vi "test_fpga_sicm_main.vi"() -> ()   [LabVIEW 2016]
uses:
  <vilib>/Platform/TimedLoop/XDataNode/timing_clust.ctl
  <vilib>/Platform/TimedLoop/XDataNode/nitl_modes.ctl
  <vilib>/Platform/TimedLoop/XDataNode/wakeup.ctl
  <vilib>/rvi/Emulation/niFpgaSctlEmulationGetInTimedLoop.vi
  <vilib>/rvi/Emulation/niFpgaEmulationReportErrorSimple.vi
  <vilib>/rvi/Emulation/niFpgaGetClockAttributes.vi
  <vilib>/rvi/Emulation/niFpgaCriticalErrorInLSC.vi
  <vilib>/Platform/TimedLoop/XDataNode/XDataNode.xnode
  <vilib>/Platform/TimedLoop/XDataNode/XDNodeRunTimeDep.lvlib
panel:
  out "sicm.Baseline":T1
  out "debug":T2
  in  "sicm.p.modes":T3
  in  "sicm.display":cluster{"sicm.ptsAfterTrig":u16}
  out "heightOut":T4
  in  "sicm.p.params":T5={"sicm.p.setPoint"=0.9999847412109375, "sicm.p.setPointFrac"=1.0, "stepDown"=0.0, "retractHeight"=0.0, "adaptiveMin"=0.0} {"sicm.p.setPoint" format="%#_3g"}
  out "sicm.triggerHeight":T6
  in  "sicm.i.current":T7
  in  "sicm.p.clocks":T8
  in  "sicm.blc.p.params":T9={"se.blc.p.postRetractDelay"=0, "se.blc.p.windowSize"=0, "se.blc.p.updateFactor"=-8, "blc.resetBackground"=FALSE}
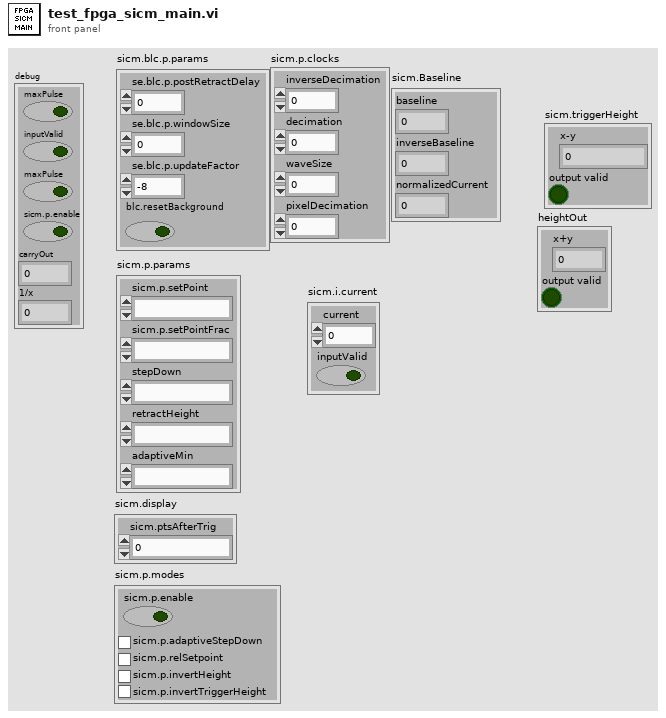
[diagram p1: front panel]
types:
  T1 = cluster{"carryOut":fxp<+/-,22,2>, "1/x":fxp<+/-,32,24>, "normalizedCurrent":fxp<+,20,1>}
  T2 = cluster{"maxPulse":bool, "inputValid":bool, "maxPulse":bool, "sicm.p.enable":bool, "carryOut":fxp<+/-,22,2>, "1/x":fxp<+/-,27,24>}
  T3 = cluster{"sicm.p.enable":bool, "sicm.p.adaptiveStepDown":bool, "sicm.p.relSetpoint":bool, "sicm.p.invertHeight":bool, "sicm.p.invertTriggerHeight":bool}
  T4 = cluster{"x+y":fxp<+/-,28,2>, "output valid":bool}
  T5 = cluster{"sicm.p.setPoint":fxp<+,20,0>, "sicm.p.setPointFrac":fxp<+/-,20,14>, "stepDown":fxp<+/-,28,4>, "retractHeight":fxp<+/-,28,4>, "adaptiveMin":fxp<+,10,0>}
  T6 = cluster{"x-y":fxp<+/-,22,4>, "output valid":bool}
  T7 = cluster{"current":fxp<+/-,24,16>, "inputValid":bool}
  T8 = cluster{"inverseDecimation":fxp<+,22,0>, "decimation":u16, "waveSize":u16, "pixelDecimation":u16}
  T9 = cluster{"se.blc.p.postRetractDelay":u16, "se.blc.p.windowSize":u16, "se.blc.p.updateFactor":i16, "blc.resetBackground":bool}
  T10 = typedef "XDNodeRunTimeDep.lvlib/timing_clust.ctl" = cluster{"Expected End [f-1]":u64, "Actual End [f-1]":u64, "Finished Late? [f-1]":bool, "Expected End [i-1]":u64, "Actual End [i-1]":u64, "Finished Late? [i-1]":bool, "Expected Start [i]":u64, "Actual Start [i]":u64, "Expected Start [f]":u64, "Actual Start [f]":u64, "Source Name":string, "Structure Name":string, "Period":i64, "Deadline":i64, "Offset":i64, "Start":i64, "Priority":i32, "Timeout":i32, "Mode":T11, "Wakeup Reason":T12, "Error":errorcluster, "Source Type":string, "Secondary Source Type":string, "Global End Time":u64, "Global Start Time":u64, "Frame Duration":u64, "Iteration Duration":u64, "Assigned CPU":i32, "I/O Scan Engine Mode":u32}
  T11 = typedef "XDNodeRunTimeDep.lvlib/nitl_modes.ctl" = enum32{"No Change", "Process missed periods, maintain original phase", "Discard missed periods, maintain original phase", "Process missed periods, ignore original phase", "Discard missed periods, ignore original phase"}
  T12 = typedef "XDNodeRunTimeDep.lvlib/wakeup.ctl" = enum32{"Normal", "Aborted", "Asynchronous wakeup", "Timing source error", "Timed loop error", "Timeout"}
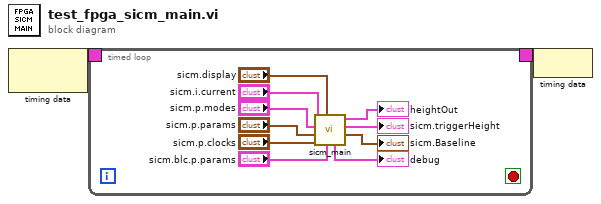
[diagram p0: block diagram]
diagram:
  n1 = node-c288() -> (w2:T10)  [unwired: 1 in]
  n2 = timed-loop {
    timing: w2 -> [_]
    timing-out: [_] -> w1
    stop <- _ stop-if-true
    n3 = call "sicm_main.vi"("sicm.blc.p.params"="sicm.blc.p.params", "sicm.display"="sicm.display", "sicm.p.clocks"="sicm.p.clocks", "sicm.p.params"="sicm.p.params", "sicm.p.modes"="sicm.p.modes", "sicm.i.current"="sicm.i.current") -> ("sicm.Baseline"=→"sicm.Baseline":T1, "sicm.triggerHeight"=→"sicm.triggerHeight":T6, "heightOut"=→"heightOut":T4, "debug"=→"debug":T2)  [unwired: 2 in]
  }
  n4 = node-c288(w1) -> ()
